vi "Subpanel Builder.vi"() -> ()   [LabVIEW 2021, in "App-Builder Library.lvlib" / "Builder.lvclass"]
uses:
  Builder.lvclass
panel:
  in  "Move Path":path
  in  "Rename files":string
  in  "Build?":bool
  in  "Next Version":string
  in  "Current Version":string
  in  "App Name":string
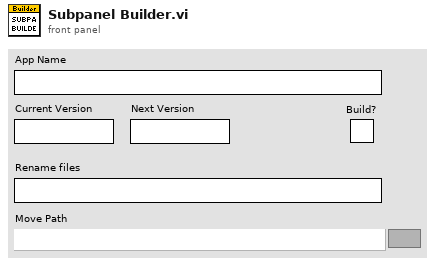
[diagram p1: front panel]
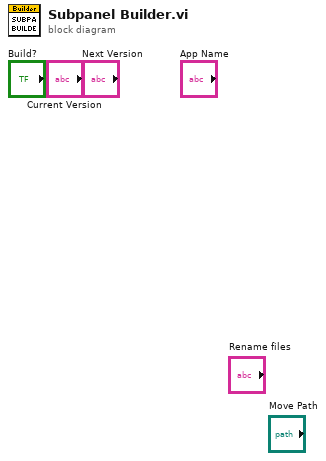
[diagram p0: block diagram]
diagram:
